vi "(SubVI) Calc. Odijk-eWLC extension.vi"(0 "dsDNA Length (bp)":dbl, 1 "nm/bp":dbl=0.338, 2 "Force (pN)":dbl, 3 "Persistence length (nm)":dbl=45.0, 4 "Elastic modulus (pN)":dbl=1200.0) -> (6 "Extension (nm)":dbl)   [LabVIEW 2014]
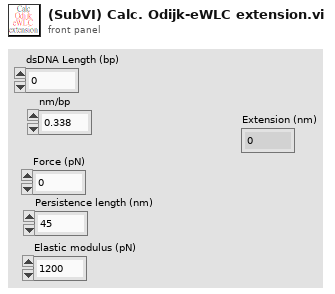
[diagram p1: front panel]
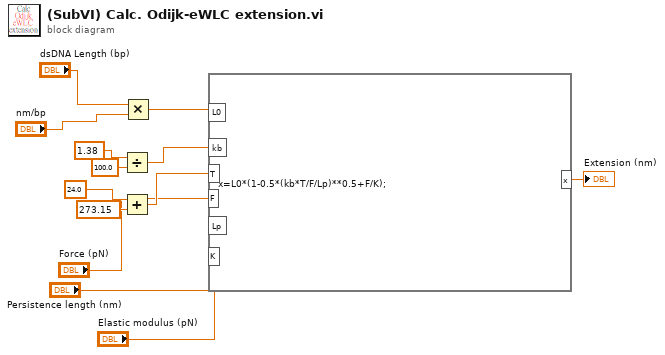
[diagram p0: block diagram]
diagram:
  n1 = Divide(x=1.38 ("input variable"), y=100.0) -> (x/y=w9:dbl)
  n2 = Add(x=24.0 ("input variable"), y=273.15) -> (x+y=w6:dbl)
  n3 = Multiply(x="dsDNA Length (bp)", y="nm/bp") -> (x*y=w12:dbl)
  n4 = formula code="x=L0*(1-0.5*(kb*T/F/Lp)**0.5+F/K);"("L0"=w12, "kb"=w9, "T"=w6, "F"="Force (pN)", "Lp"="Persistence length (nm)", "K"="Elastic modulus (pN)") -> ("x"=→"Extension (nm)":dbl)
